vi "LVClass_ModalCoef GetTypePhase.vi"(0 "ModalCoef in":refnum<class "ModalCoef.lvclass">, 11 "error in (no error)":errorcluster) -> (4 "ModalCoef out":refnum<class "ModalCoef.lvclass">, 6 "TypePhase":T1, 15 "error out":errorcluster)   [LabVIEW 2020, in "ModalCoef.lvclass"]
doc: "Get preferences for phase reconstruction from Zernike decomposition.\n\n--------------------------------------------------------------------------------\n\n<B>ComputePhaseSetIn </B> : ComputePhaseSet object.\n<B>ComputePhaseSetOut </B> : ComputePhaseSet object.\n<B>normalisation </B> : Normalisation Phase coefficients enumeration :\n * 0 : standard\n * 1 : rms\n<B>nb_coeffs_total </B> : Number of the Zernike coefficients used in the polynomial base.\n<B>nb_coeffs_to_filter </B> : Number of the Zernike coefficients to filter in the polynomial base.\n<B>coeffs_to_filter </B> : Indices of the Zernike coefficients to filter in the polynomial base.\n<B>projection_pupil_center </B> : Center of the projection pupil, in number of subpupils.\n<B>projection_pupil_radius </B> : Projection pupil radius, in number of subpupils.\n<B>ErrorIn </B> : Error\n<B>ErrorOut </B> : Error\n\n--------------------------------------------------------------------------------"
uses:
  ModalCoef.lvclass
  WavefrontModalReconstructionType.ctl
  ModalCoef.lvclass/ModalCoef.ctl
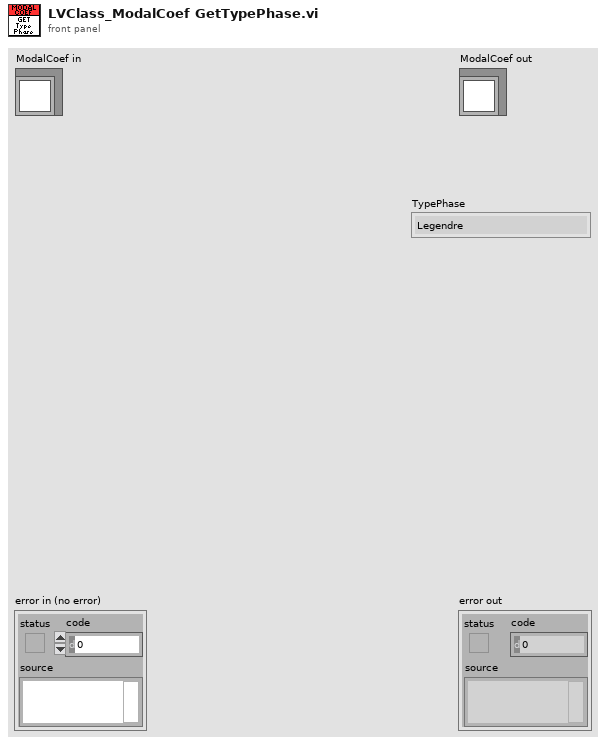
[diagram p1: front panel]
types:
  T1 = typedef "WavefrontModalReconstructionType.ctl" = enum16{"Legendre", "Zernike"}
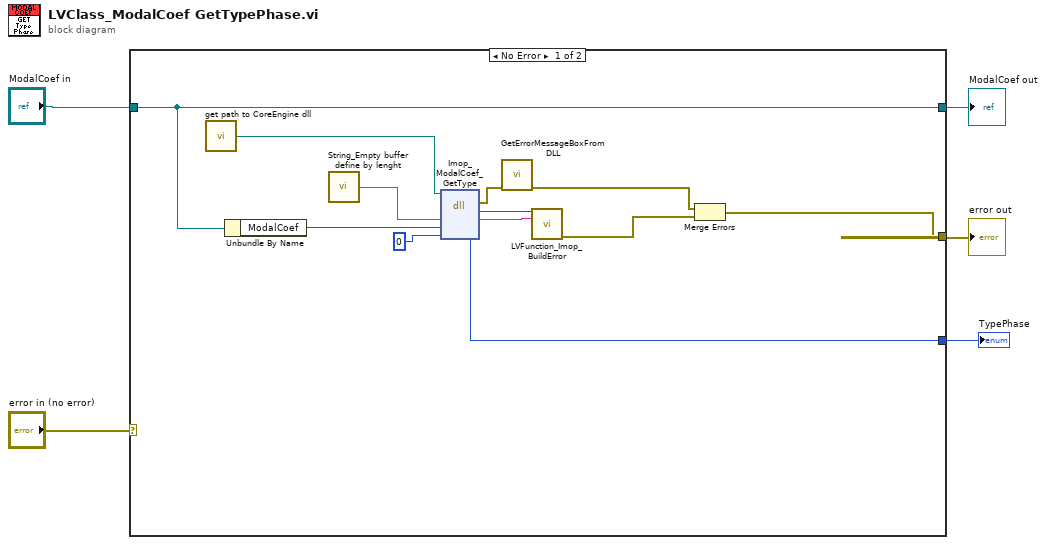
[diagram p0: block diagram]
diagram:
  n1 = case shown="No Error" "error in (no error)" {
    selector: "error in (no error)" -> [_ w19]
    tunnel: [w7 w19] -> w2
    tunnel: [w11 w18] -> w4
    tunnel: "ModalCoef in" -> [w11 w18]
    tunnel: [w6 _] -> w1
    frame No Error {
      n2 = call "get path to CoreEngine dll.vi"() -> ("path to c_interface_vc100.dll"=w14:path)  [unwired: 12 in, 3 out]
      n3 = Unbundle By Name(w11) -> ("ModalCoef"=w10:i32)
      n4 = call "String_Empty buffer define by lenght.vi"() -> ("Empty buffer"=w15:string)  [unwired: 1 in]
      n5 = dll-call lib="D:/2_trunk/Soft_haso/ImOpCoreEngine4_LV2011/DLLs/ImopEngine4_vc100.dll" fn="Imop_ModalCoef_GetType"(path in=w14, "message"=w15, "objet"=w10, "TypePhase"=u8 0 ("normalisation")) -> (error out=w13:errorcluster, "return type"=w17:i32, "message"=w16:string, "TypePhase"=w6:u8)  [unwired: 3 in, 1 out]
      n6 = call "GetErrorMessageBoxFromDLL.vi"("error IN"=w13) -> ("error OUT"=w9:errorcluster)  [unwired: 10 in]
      n7 = call "LVFunction_Imop_BuildError.vi"("code"=w17, "String to Prepend to source (\"\")"=w16) -> ("error out"=w8:errorcluster)  [unwired: 13 in]
      n8 = Merge Errors(w9, w8) -> (w7:errorcluster)
    }
    frame Error {
    }
  }
  "error out" <- w2
  "ModalCoef out" <- w4
  "TypePhase" <- w1
